vi "CRYGraph Main.vi"() -> ()   [LabVIEW 2013]
uses:
  Control/SplitterBar.ctl
  <vilib>/Utility/inputDevices.llb/closeMouse.vi
  CRYNew View Global.vi
  CRYView Global.vi
  <vilib>/Utility/inputDevices.llb/mouseAcquire.vi
  SubVI/CRYMain Sub Window Global.vi
  <vilib>/Utility/cursorutil.llb/Set Cursor (Icon Pict).vi
panel:
  in  "bWaitCommand":bool
  in  "Docking Start":bool
  in  "nIDV":i32=10
  in  "pSPRefParent":refnum<vi>
  in  "pVIRefParent":refnum<vi>
  in  "sViewName":string="DataView"
  out "Index":i32
  in  "stop":bool
  out "StateOut":bool
  out "Bar_shadow":bool
  in  "Resize FrontPanel":bool
  in  "Add Top":bool
  in  "Add Left":bool
  out "s2":T1
  out "s30":T1
  out "s29":T1
  out "s28":T1
  out "s27":T1
  out "s26":T1
  out "s25":T1
  in  "Mouse Pos":T2
  in  "ToolbarClicked":bool
  in  "Add Bottom":bool
  in  "activated_idx":i32
  in  "close_panel":bool=TRUE
  in  "Resize_Panels":bool
  in  "splitter_down_flag":bool=TRUE
  in  "spliter_index":i32
  out "s7":T1
  out "s1":T1
  out "s12":T1
  out "s5":T1
  out "s6":T1
  out "s11":T1
  out "s10":T1
  out "s19":T1
  out "s9":T1
  out "s8":T1
  out "s24":T1
  out "s23":T1
  out "s22":T1
  out "s21":T1
  out "s20":T1
  out "s18":T1
  out "s17":T1
  out "s16":T1
  out "s15":T1
  out "s14":T1
  out "s13":T1
  out "s4":T1
  out "s3":T1
  in  "Add Right":bool
types:
  T1 = typedef "SplitterBar.ctl" = bool
  T2 = cluster{"Horizontal":i32, "Vertical":i32, "Scrolling":i32}
  T3 = cluster{"Ctrl Reference":refnum<vi>, "bObjMove":bool, "Position_top":i32, "Position_objtop":i32, "isVertical":bool, "Position_left":i32, "Position_objleft":i32}
  T4 = cluster{"sAction":string, "sType":string, "sQueueName":string, "sGraphName":string, "sData":string, "nData":i32, "pVIRef":refnum<vi>, "pSPRef":refnum<vi>}
  T5 = cluster{"TitlebarActiveColor Graph":u32, "TitlebarActiveColor Graph 2":u32}[]
  T6 = typedef "Graph Main Info Cluster.ctl" = cluster{"Selected_BarIdx":i32, "Selected_PanelIdx":i32, "Graph Main VIRef":refnum<vi>, "ToolBarClick":bool, "Spliter Ref Array":refnum<vi>[], "Panel Ref Array":refnum<vi>[], "Spliter_matrix":i32[][], "Panel_matrix":i32[][], "child_spliterIdx_matrix":i32[][], "split_pos_matrix":i32[][], "Title State":bool, "sQueueName":string, "Frame nID":i32, "Graph VIRef Array":cluster{"Graph VIRef":refnum<vi>, "Panel Idx":i32, "Frame VIRef":refnum<vi>, "Icon Ring":i32, "Graph Type":string}[], "View Type":string}
  T7 = cluster{"nID":i32, "sName":string, "sType":string, "sProperty":string, "sTemplet":string, "sDocking":string, "pVIRef":refnum<vi>, "pSPRef":refnum<vi>, "pRefTemplet":refnum<vi>, "pRefSplitter":refnum<vi>[], "nPosSplitter":i32[], "pRefSP":refnum<vi>[], "nSPID":i32[], "sSPDock":string[], "nIDFrame":i32[], "nIDPanel":i32[], "nActiveFrame":i32, "nCountFrame":i32, "cFrame":cluster{"nID":i32, "sName":string, "sType":string, "sTitle":string, "sIcon":string, "pVIRef":refnum<vi>, "pSPRef":refnum<vi>, "cWin":cluster{"sName":string, "sType":string, "pVIRef":refnum<vi>, "sData":string}, "cTab":cluster{"sTitle":string, "sIcon":string, "pSpliter":refnum<vi>, "nAvtivePage":i32, "nIDPage":i32[], "nIDFrame":i32[]}, "sData":string}[], "sData":string, "sSplitterName":string[]}
  T8 = cluster{"sCmdType":string, "nIDView":i32, "sAction":string, "sData":string, "sOption":string, "nData":i32, "nOption":i32, "pVIRef":refnum<vi>, "pSPRef":refnum<vi>, "bWaitRef":refnum<vi>, "Result":variant}
  T9 = cluster{"button 1":bool, "button 2":bool, "button 3":bool, "button 4":bool}
  T10 = typedef "LVRectTypeDef.ctl" = cluster{"Left":i16, "Top":i16, "Right":i16, "Bottom":i16}
  T11 = cluster{"Left":bool, "Top":bool, "Right":bool, "Bottom":bool}
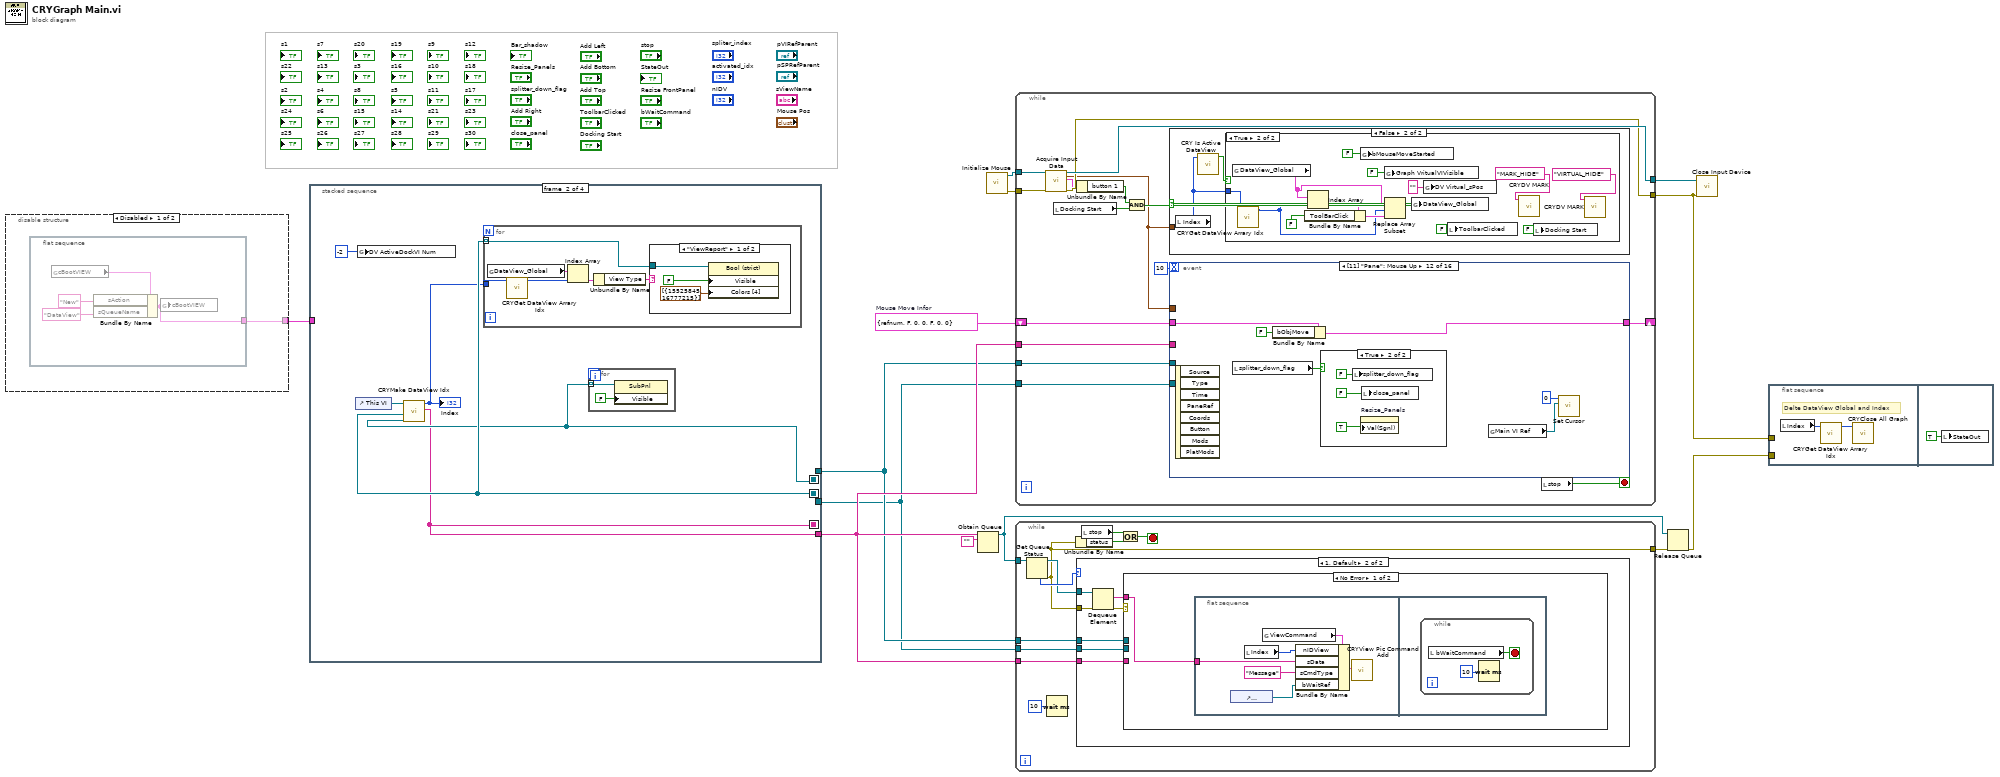
[diagram p0: block diagram]
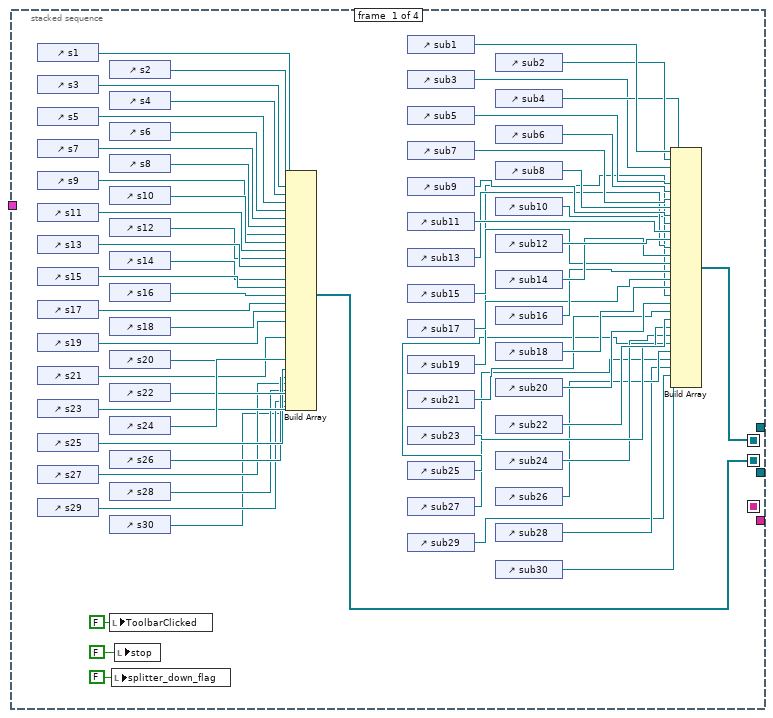
[diagram p3: hidden frame]
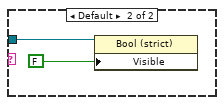
[diagram p4: hidden frame]
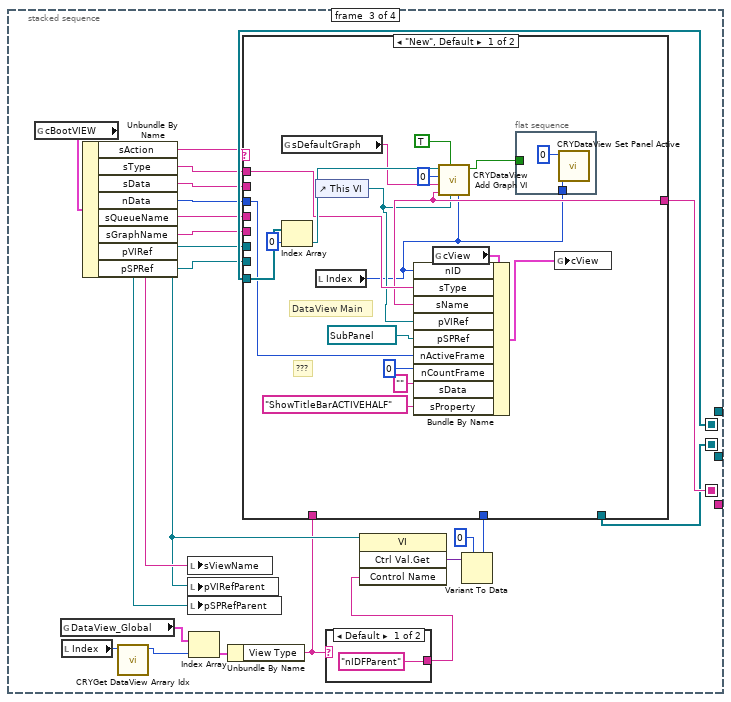
[diagram p5: hidden frame]
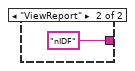
[diagram p6: hidden frame]
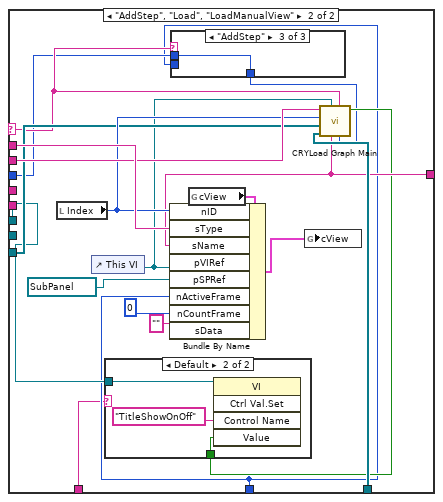
[diagram p7: hidden frame]
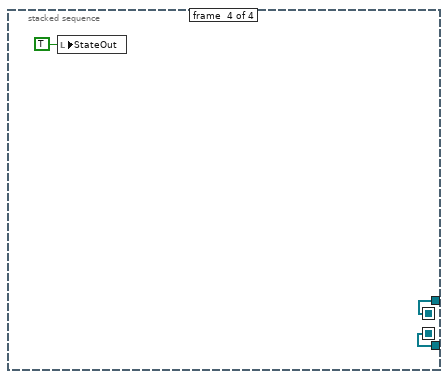
[diagram p11: hidden frame]
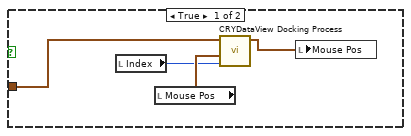
[diagram p14: hidden frame]
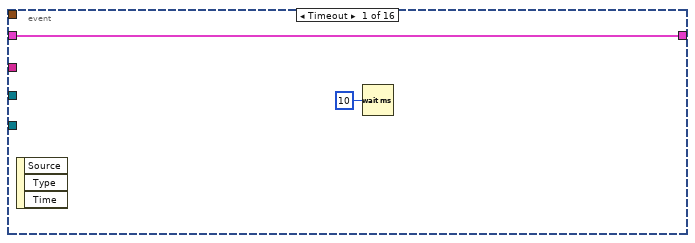
[diagram p16: hidden frame]
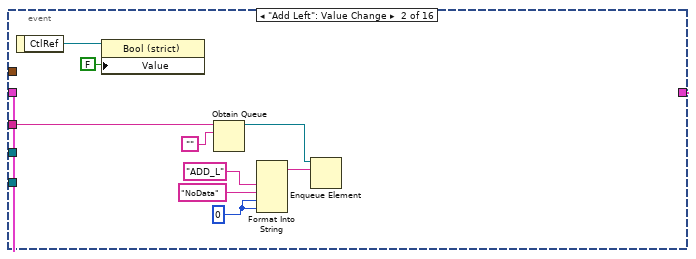
[diagram p17: hidden frame]
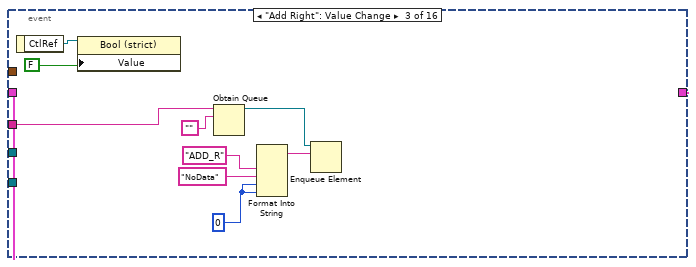
[diagram p18: hidden frame]
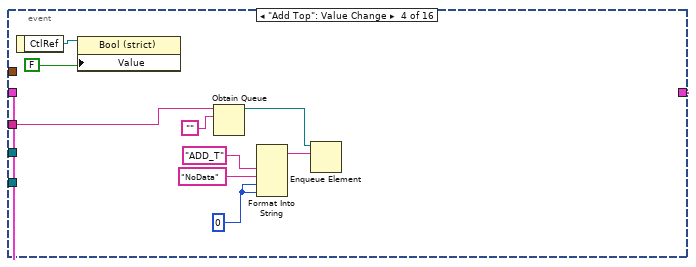
[diagram p19: hidden frame]
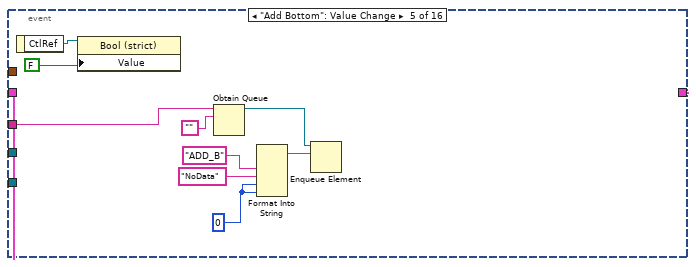
[diagram p20: hidden frame]
diagram:
  w13 = T3 {"Ctrl Reference"=refnum, "bObjMove"=FALSE, "Position_top"=0, "Position_objtop"=0, "isVertical"=FALSE, "Position_left"=0, "Position_objleft"=0}  # Mouse Move Infor
  n1 = disable-structure shown="Disabled" {
    disable-tunnel: [w14 _] -> w4
    frame Disabled {
      n2 = flat-sequence {
        tunnel: [w15] -> w14
        frame #0 {
          n3 = global read "CRYView Global.vi" "cBootVIEW"() -> (w18:T4)
          n4 = Bundle By Name(cluster=w18, "sAction"="New", "sQueueName"="DataView") -> (w15:T4)
          n5 = global write "CRYView Global.vi" "cBootVIEW"(w15) -> ()
        }
      }
    }
    frame Enabled {
    }
  }
  n6 = stacked-sequence {
    seq-local: [w22 _ _ _] -> [_ w88 w113 w171]
    seq-local: [w45 _ _ _] -> [_ w87 w122 w172]
    seq-local: [_ w86 _ _] -> [_ _ w123 _]
    tunnel: [_ w86 _ _] -> w5
    tunnel: w4 -> [_ _ _ _]
    tunnel: [_ _ _ w171] -> w1
    tunnel: [_ _ _ w172] -> w3
    frame #0 {
      n7 = control-ref of="s1"() -> (w24:refnum<vi>)
      n8 = control-ref of="s3"() -> (w46:refnum<vi>)
      n9 = control-ref of="s5"() -> (w48:refnum<vi>)
      n10 = control-ref of="s7"() -> (w50:refnum<vi>)
      n11 = control-ref of="s9"() -> (w52:refnum<vi>)
      n12 = control-ref of="s11"() -> (w54:refnum<vi>)
      n13 = control-ref of="s13"() -> (w56:refnum<vi>)
      n14 = control-ref of="s15"() -> (w58:refnum<vi>)
      n15 = control-ref of="s17"() -> (w60:refnum<vi>)
      n16 = control-ref of="s19"() -> (w62:refnum<vi>)
      n17 = control-ref of="s21"() -> (w64:refnum<vi>)
      n18 = control-ref of="s23"() -> (w66:refnum<vi>)
      n19 = control-ref of="s25"() -> (w31:refnum<vi>)
      n20 = control-ref of="s27"() -> (w29:refnum<vi>)
      n21 = control-ref of="s29"() -> (w27:refnum<vi>)
      n22 = control-ref of="s2"() -> (w23:refnum<vi>)
      n23 = control-ref of="s4"() -> (w47:refnum<vi>)
      n24 = control-ref of="s6"() -> (w49:refnum<vi>)
      n25 = control-ref of="s8"() -> (w51:refnum<vi>)
      n26 = control-ref of="s10"() -> (w53:refnum<vi>)
      n27 = control-ref of="s12"() -> (w55:refnum<vi>)
      n28 = control-ref of="s14"() -> (w57:refnum<vi>)
      n29 = control-ref of="s16"() -> (w59:refnum<vi>)
      n30 = control-ref of="s18"() -> (w61:refnum<vi>)
      n31 = control-ref of="s20"() -> (w63:refnum<vi>)
      n32 = control-ref of="s22"() -> (w65:refnum<vi>)
      n33 = control-ref of="s24"() -> (w67:refnum<vi>)
      n34 = control-ref of="s26"() -> (w30:refnum<vi>)
      n35 = control-ref of="s28"() -> (w28:refnum<vi>)
      n36 = control-ref of="s30"() -> (w26:refnum<vi>)
      n37 = local write "ToolbarClicked"(FALSE ("ToolbarClicked")) -> ()
      n38 = local write "splitter_down_flag"(FALSE ("m_down_flag")) -> ()
      n39 = local write "stop"(FALSE ("stop")) -> ()
      n40 = Build Array(w24, w23, w46, w47, w48, w49, w50, w51, w52, w53, w54, w55, w56, w57, w58, w59, w60, w61, w62, w63, w64, w65, w66, w67, w31, w30, w29, w28, w27, w26) -> (w22:refnum<vi>[])
      n41 = control-ref of="sub1"() -> (w83:refnum<vi>)
      n42 = control-ref of="sub3"() -> (w25:refnum<vi>)
      n43 = control-ref of="sub5"() -> (w80:refnum<vi>)
      n44 = control-ref of="sub7"() -> (w78:refnum<vi>)
      n45 = control-ref of="sub9"() -> (w76:refnum<vi>)
      n46 = control-ref of="sub11"() -> (w75:refnum<vi>)
      n47 = control-ref of="sub13"() -> (w73:refnum<vi>)
      n48 = control-ref of="sub15"() -> (w71:refnum<vi>)
      n49 = control-ref of="sub17"() -> (w69:refnum<vi>)
      n50 = control-ref of="sub19"() -> (w43:refnum<vi>)
      n51 = control-ref of="sub21"() -> (w41:refnum<vi>)
      n52 = control-ref of="sub23"() -> (w39:refnum<vi>)
      n53 = control-ref of="sub25"() -> (w37:refnum<vi>)
      n54 = control-ref of="sub27"() -> (w35:refnum<vi>)
      n55 = control-ref of="sub29"() -> (w33:refnum<vi>)
      n56 = control-ref of="sub2"() -> (w82:refnum<vi>)
      n57 = control-ref of="sub4"() -> (w81:refnum<vi>)
      n58 = control-ref of="sub6"() -> (w79:refnum<vi>)
      n59 = control-ref of="sub8"() -> (w77:refnum<vi>)
      n60 = control-ref of="sub10"() -> (w68:refnum<vi>)
      n61 = control-ref of="sub12"() -> (w74:refnum<vi>)
      n62 = control-ref of="sub14"() -> (w72:refnum<vi>)
      n63 = control-ref of="sub16"() -> (w70:refnum<vi>)
      n64 = control-ref of="sub18"() -> (w44:refnum<vi>)
      n65 = control-ref of="sub20"() -> (w42:refnum<vi>)
      n66 = control-ref of="sub22"() -> (w40:refnum<vi>)
      n67 = control-ref of="sub24"() -> (w38:refnum<vi>)
      n68 = control-ref of="sub26"() -> (w36:refnum<vi>)
      n69 = control-ref of="sub28"() -> (w34:refnum<vi>)
      n70 = control-ref of="sub30"() -> (w32:refnum<vi>)
      n71 = Build Array(w83, w82, w25, w81, w80, w79, w78, w77, w76, w68, w75, w74, w73, w72, w71, w70, w69, w44, w43, w42, w41, w40, w39, w38, w37, w36, w35, w34, w33, w32) -> (w45:refnum<vi>[])
    }
    frame #1 {
      n72 = control-ref of="This VI"() -> (w89:refnum<vi>)
      n73 = global write "CRYNew View Global.vi" "DV ActiveDockVI Num"(-2 ("DV ActiveDockVI Num")) -> ()
      n74 = call "CRYMake DataView Idx.vi"("Panel Ref Array"=w87, "Spliter Ref Array"=w88, "VI Ref"=w89) -> ("sQueueName Out"=w86:string, "New DataView Idx"=w85:i32)  [unwired: 7 in]
      "Index" <- w85
      n75 = for {
        tunnel: w88 -> [w97] mode=indexing
        tunnel: w85 -> [w93]
        n76 = global read "CRYNew View Global.vi" "DataView_Global"() -> (w96:T6[])
        n77 = call "CRYGet DataView Arrary Idx.vi"("DataView Idx In"=w93) -> ("DataView Arrary Idx out"=w94:i32)  [unwired: 10 in]
        n78 = Index Array(array=w96, index=w94) -> (element=w95:T6)
        n79 = Unbundle By Name(w95) -> ("View Type"=w92:string)
        n80 = case shown="\"ViewReport\"" w92 {
          tunnel: w97 -> [w99 w101]
          frame "ViewReport" {
            n81 = property class="Bool (strict)"(reference=w99, "Visible"=FALSE, "Colors [4]"=T5 [{"TitlebarActiveColor Graph"=15525845, "TitlebarActiveColor Graph 2"=16777215}]) -> ()  [unwired: 1 in, 2 out]
          }
          frame Default {
            n82 = property class="Bool (strict)"(reference=w101, "Visible"=FALSE) -> ()  [unwired: 1 in, 2 out]
          }
        }
      }
      n83 = for {
        tunnel: w87 -> [w90] mode=indexing
        n84 = property class="SubPnl"(reference=w90, "Visible"=FALSE) -> ()  [unwired: 1 in, 2 out]
      }
    }
    frame #2 {
      n85 = global read "CRYView Global.vi" "cBootVIEW"() -> (w121:T4)
      n86 = global read "CRYNew View Global.vi" "DataView_Global"() -> (w108:T6[])
      n87 = local read "Index"() -> (w107:i32)
      n88 = Unbundle By Name(w121) -> ("sAction"=w117:string, "sType"=w116:string, "sData"=w119:string, "nData"=w118:i32, "sQueueName"=w115:string, "sGraphName"=w120:string, "pVIRef"=w109:refnum<vi>, "pSPRef"=w114:refnum<vi>)
      n89 = call "CRYGet DataView Arrary Idx.vi"("DataView Idx In"=w107) -> ("DataView Arrary Idx out"=w103:i32)  [unwired: 10 in]
      n90 = local write "sViewName"(w115) -> ()
      n91 = local write "pVIRefParent"(w109) -> ()
      n92 = local write "pSPRefParent"(w114) -> ()
      n93 = Index Array(array=w108, index=w103) -> (element=w106:T6)
      n94 = Unbundle By Name(w106) -> ("View Type"=w104:string)
      n95 = case shown="Default" w104 {
        tunnel: ["nIDFParent" ("Control Name") "nIDF" ("Control Name")] -> w105
        frame Default {
        }
        frame "ViewReport" {
        }
      }
      n96 = invoke class="VI" method="Ctrl Val.Get"(reference=w109, "Control Name"=w105) -> ("Get Control Value Variant"=w112:variant)  [unwired: 2 in, 3 out]
      n97 = Variant To Data(type=0 ("nIDFParent"), Variant=w112) -> (data=w110:i32)  [unwired: 1 in, 1 out]
      n98 = case shown="\"New\", Default" w117 {
        selector: w117 -> [_ w151]
        tunnel: w115 -> [_ _]
        tunnel: w120 -> [_ _]
        tunnel: w119 -> [_ w158]
        tunnel: w118 -> [w127 w150]
        tunnel: w109 -> [_ w148]
        tunnel: w114 -> [_ _]
        tunnel: w116 -> [w133 w164]
        tunnel: w123 -> [w132 w153]
        tunnel: w122 -> [w143 w156]
        tunnel: w113 -> [_ w155]
        tunnel: w110 -> [_ w147]
        tunnel: w104 -> [_ w146]
        frame "New", Default {
          # "DataView Main"
          # "???"
          n99 = global read "CRYView Global.vi" "sDefaultGraph"() -> (w134:string)
          n100 = Index Array(array=w143, index=0) -> (element=w141:refnum<vi>)
          n101 = control-ref of="This VI"() -> (w129:refnum<vi>)
          n102 = local read "Index"() -> (w126:i32)
          n103 = global read "CRYView Global.vi" "cView"() -> (w135:T7)
          n104 = Bundle By Name(cluster=w135, "nID"=w126, "sType"=w133, "sName"=w132, "pVIRef"=w129, "pSPRef"=refnum<vi> refnum, "nActiveFrame"=w127, "nCountFrame"=0 ("nActiveFrame"), "sData"="", "sProperty"="ShowTitleBarACTIVEHALF") -> (w130:T7)
          n105 = call "CRYDataView Add Graph VI.vi"("DataView Idx"=w126, "Graph Main VIRef In"=w129, "isFirstPanel"=TRUE, "Queue Name"=w132, "GraphType"=w134, "panel_index"=0, "Panel Ref In"=w141) -> ("bResult"=w128:bool)  [unwired: 4 in]
          n106 = flat-sequence {
            tunnel: w126 -> [w145]
            tunnel: w128 -> [_]
            frame #0 {
              n107 = call "CRYDataView Set Panel Active.vi"("DataView Index"=w145, "Selected Panel Idx In"=0) -> ()  [unwired: 10 in]
            }
          }
          n108 = global write "CRYView Global.vi" "cView"(w130) -> ()
        }
        frame "AddStep", "Load", "LoadManualView" {
          n109 = local read "Index"() -> (w157:i32)
          n110 = control-ref of="This VI"() -> (w154:refnum<vi>)
          n111 = case shown="\"AddStep\"" w151 {
            tunnel: w147 -> [_ w169 _]
            tunnel: [w168 w169 w170] -> w149
            tunnel: w150 -> [w168 _ w170]
            frame "LoadManualView", Default {
            }
            frame "Load" {
            }
            frame "AddStep" {
            }
          }
          n112 = global read "CRYView Global.vi" "cView"() -> (w163:T7)
          n113 = Bundle By Name(cluster=w163, "nID"=w157, "sType"=w164, "sName"=w153, "pVIRef"=w154, "pSPRef"=refnum<vi> refnum, "nActiveFrame"=w147, "nCountFrame"=0 ("nActiveFrame"), "sData"="") -> (w159:T7)
          n114 = global write "CRYView Global.vi" "cView"(w159) -> ()
          n115 = call "CRYLoad Graph Main.vi"("nData"=w149, "sAction"=w151, "sQueue Name"=w153, "Graph Main Ref"=w154, "Spliter Ref Array"=w155, "Panel Ref Array"=w156, "DataView Index"=w157, "Flattend Data"=w158) -> ("Title State"=w152:bool)  [unwired: 3 in]
          n116 = case shown="Default" w146 {
            tunnel: w152 -> [_ w166]
            tunnel: w148 -> [_ w165]
            frame "ViewReport" {
            }
            frame Default {
              n117 = invoke class="VI" method="Ctrl Val.Set"(reference=w165, "Control Name"="TitleShowOnOff" ("Resize Panel Str"), "Value"=w166) -> ()  [unwired: 2 in, 5 out]
            }
          }
        }
      }
    }
    frame #3 {
      n118 = local write "StateOut"(TRUE ("StateOut")) -> ()
    }
  }
  n119 = Obtain Queue(name (unnamed)=w5, element data type="") -> (queue out=w11:refnum<queue>)  [unwired: 3 in, 2 out]
  n120 = call <vilib>:"Initialize Mouse.vi"() -> ("error out"=w9:errorcluster, "device ID"=w10:refnum<k1>)  [unwired: 10 in]
  n121 = while {
    tunnel: w11 -> [w183]
    tunnel: w1 -> [w180]
    tunnel: w3 -> [w179]
    tunnel: [w178] -> w7
    tunnel: w5 -> [w174]
    stop <- w175 stop-if-true
    n122 = Get Queue Status(queue=w183) -> (queue out=w181:refnum<queue>, error out=w178:errorcluster, # elements in queue=w182:i32)  [unwired: 2 in, 5 out]
    n123 = Wait (ms)(milliseconds to wait=u32 10) -> ()  [unwired: 1 out]
    n124 = Unbundle By Name(w178) -> ("status"=w177:bool)
    n125 = case shown="1, Default" w182 {
      tunnel: w178 -> [_ w187]
      tunnel: w181 -> [_ w191]
      tunnel: w180 -> [_ w189]
      tunnel: w179 -> [_ w188]
      tunnel: w174 -> [_ w185]
      frame 0 {
      }
      frame 1, Default {
        n126 = Dequeue Element(queue=w191, error in (no error)=w187) -> (element=w190:string, error out=w186:errorcluster)  [unwired: 1 in, 2 out]
        n127 = case shown="No Error" w186 {
          tunnel: w190 -> [w192 _]
          tunnel: w189 -> [_ _]
          tunnel: w188 -> [_ _]
          tunnel: w185 -> [_ _]
          frame No Error {
            n128 = flat-sequence {
              tunnel: w192 -> [w196]
              frame #0 {
                n129 = control-ref of="bWaitCommand"() -> (w195:refnum<vi>)
                n130 = local read "Index"() -> (w193:i32)
                n131 = global read "CRYView Global.vi" "ViewCommand"() -> (w194:T8)
                n132 = Bundle By Name(cluster=w194, "nIDView"=w193, "sData"=w196, "sCmdType"="Message" ("sAction"), "bWaitRef"=w195) -> (w197:T8)
                n133 = call "CRYView Pic Command Add.vi"("cCommand"=w197) -> ()  [unwired: 11 in]
              }
              frame #1 {
                n134 = while {
                  stop <- w200 stop-if-true
                  n135 = local read "bWaitCommand"() -> (w200:bool)
                  n136 = Wait (ms)(milliseconds to wait=u32 10) -> ()  [unwired: 1 out]
                }
              }
            }
          }
          frame Error {
          }
        }
      }
    }
    n137 = local read "stop"() -> (w176:bool)
    n138 = Or(x=w176, y=w177) -> (x .or. y?=w175:bool)
  }
  n139 = while {
    tunnel: w3 -> [w202]
    shift-right: [w214] -> _
    shift-left: w13 -> [w216]
    tunnel: w1 -> [w215]
    tunnel: w5 -> [w213]
    tunnel: w10 -> [w212]
    tunnel: w9 -> [w211]
    tunnel: [w210] -> w8
    tunnel: [w209] -> w2
    stop <- w201 stop-if-true
    n140 = call-poly <vilib>:"Acquire Input Data.vi"("device ID"=w212, "error in (no error)"=w211) -> ("device ID"=w210:refnum<k1>, "axis info"=w203:T2, "button info"=w208:T9, "error out"=w209:errorcluster)  [unwired: 14 in]
    n141 = local read "Docking Start"() -> (w206:bool)
    n142 = Unbundle By Name(w208) -> ("button 1"=w205:bool)
    n143 = And(x=w205, y=w206) -> (x .and. y?=w204:bool)
    n144 = case shown="False" w204 {
      tunnel: w203 -> [w220 _]
      frame True {
        n145 = local read "Index"() -> (w217:i32)
        n146 = local read "Mouse Pos"() -> (w219:T2)
        n147 = call "CRYDataView Docking Process.vi"("DataView Index"=w217, "Start Pos"=w219, "Mouse Pos"=w220) -> ("StartPositin Out"=w218:T2)  [unwired: 8 in]
        n148 = local write "Mouse Pos"(w218) -> ()
      }
      frame False {
        n149 = local read "Index"() -> (w222:i32)
        n150 = call "CRY Is Active DataView.vi"("DataView Index"=w222) -> ("bResult"=w221:bool)  [unwired: 10 in]
        n151 = case shown="True" w221 {
          tunnel: w222 -> [_ w227]
          frame False {
          }
          frame True {
            n152 = global read "CRYNew View Global.vi" "DataView_Global"() -> (w232:T6[])
            n153 = call "CRYGet DataView Arrary Idx.vi"("DataView Idx In"=w227) -> ("DataView Arrary Idx out"=w226:i32)  [unwired: 10 in]
            n154 = Index Array(array=w232, index=w226) -> (element=w235:T6)
            n155 = Bundle By Name(cluster=w235, "ToolBarClick"=FALSE) -> (w234:T6)
            n156 = global write "CRYNew View Global.vi" "bMouseMoveStarted"(FALSE ("VritualVIVisible")) -> ()
            n157 = global write "CRYNew View Global.vi" "Graph VritualVIVisible"(FALSE ("VritualVIVisible")) -> ()
            n158 = Replace Array Subset(array=w232, new element=w234, index=w226) -> (w236:T6[])
            n159 = global write "CRYNew View Global.vi" "DataView_Global"(w236) -> ()
            n160 = global write "CRYNew View Global.vi" "DV Virtual_sPos"("" ("DV Virtual_sPos")) -> ()
            n161 = local write "ToolbarClicked"(FALSE ("ToolbarClicked")) -> ()
            n162 = call "CRYDV MARK.vi"("sAction"="MARK_HIDE") -> ()  [unwired: 9 in, 1 out]
            n163 = local write "Docking Start"(FALSE ("Docking Start")) -> ()
            n164 = call "CRYDV MARK.vi"("sAction"="VIRTUAL_HIDE") -> ()  [unwired: 9 in, 1 out]
          }
        }
      }
    }
    n165 = event shown="[11] \"Pane\": Mouse Up" {
      selector: _ -> [_ _ _ _ _ _ _ _ _ _ _ _ _ _ _ _]
      dyn-events: _ -> [_ _ _ _ _ _ _ _ _ _ _ _ _ _ _ _]
      timeout: 10 -> [_ _ _ _ _ _ _ _ _ _ _ _ _ _ _ _]
      tunnel: w202 -> [_ _ _ _ _ _ _ _ _ w291 _ _ _ _ _ _]
      tunnel: w216 -> [w237 w246 w256 w266 w276 w281 w284 w288 _ _ w306 w313 w322 w338 _ _]
      tunnel: [w237 w246 w256 w266 w276 w281 w284 w288 _ _ w305 w315 w324 w339 _ _] -> w214
      tunnel: w215 -> [_ _ _ _ _ _ _ _ _ _ _ _ _ _ _ _]
      tunnel: w213 -> [_ w239 w249 w259 w269 _ _ _ _ _ _ _ _ w331 _ _]
      tunnel: w203 -> [_ _ _ _ _ _ _ w287 w289 w292 w307 _ _ _ _ _]
      event Timeout {
        n166 = event-data() -> ()  [unwired: 1 in, 3 out]
        n167 = Wait (ms)(milliseconds to wait=u32 10) -> ()  [unwired: 1 out]
      }
      event "Add Left": Value Change {
        w240 = 0 ("input 3")
        n168 = event-data() -> ("CtlRef"=w248:refnum<vi>)  [unwired: 1 in]
        n169 = property class="Bool (strict)"(reference=w248, "Value"=FALSE) -> ()  [unwired: 1 in, 2 out]
        n170 = Obtain Queue(name (unnamed)=w239, element data type="") -> (queue out=w242:refnum<queue>)  [unwired: 3 in, 2 out]
        n171 = Format Into String("ADD_L" ("input 1"), "NoData" ("input 2"), w240, w240) -> (resulting string=w241:string)  [unwired: 3 in, 1 out]
        n172 = Enqueue Element(queue=w242, element=w241) -> ()  [unwired: 1 in, 4 out]
      }
      event "Add Right": Value Change {
        w250 = 0 ("input 3")
        n173 = event-data() -> ("CtlRef"=w258:refnum<vi>)  [unwired: 1 in]
        n174 = property class="Bool (strict)"(reference=w258, "Value"=FALSE) -> ()  [unwired: 1 in, 2 out]
        n175 = Obtain Queue(name (unnamed)=w249, element data type="") -> (queue out=w252:refnum<queue>)  [unwired: 3 in, 2 out]
        n176 = Format Into String("ADD_R" ("input 1"), "NoData" ("input 2"), w250, w250) -> (resulting string=w251:string)  [unwired: 3 in, 1 out]
        n177 = Enqueue Element(queue=w252, element=w251) -> ()  [unwired: 1 in, 4 out]
      }
      event "Add Top": Value Change {
        w260 = 0 ("input 3")
        n178 = event-data() -> ("CtlRef"=w268:refnum<vi>)  [unwired: 1 in]
        n179 = property class="Bool (strict)"(reference=w268, "Value"=FALSE) -> ()  [unwired: 1 in, 2 out]
        n180 = Obtain Queue(name (unnamed)=w259, element data type="") -> (queue out=w262:refnum<queue>)  [unwired: 3 in, 2 out]
        n181 = Format Into String("ADD_T" ("input 1"), "NoData" ("input 2"), w260, w260) -> (resulting string=w261:string)  [unwired: 3 in, 1 out]
        n182 = Enqueue Element(queue=w262, element=w261) -> ()  [unwired: 1 in, 4 out]
      }
      event "Add Bottom": Value Change {
        w270 = 0 ("input 3")
        n183 = event-data() -> ("CtlRef"=w278:refnum<vi>)  [unwired: 1 in]
        n184 = property class="Bool (strict)"(reference=w278, "Value"=FALSE) -> ()  [unwired: 1 in, 2 out]
        n185 = Obtain Queue(name (unnamed)=w269, element data type="") -> (queue out=w272:refnum<queue>)  [unwired: 3 in, 2 out]
        n186 = Format Into String("ADD_B" ("input 1"), "NoData" ("input 2"), w270, w270) -> (resulting string=w271:string)  [unwired: 3 in, 1 out]
        n187 = Enqueue Element(queue=w272, element=w271) -> ()  [unwired: 1 in, 4 out]
      }
      event Mouse Enter {
        # "Splitter Mouse Enter"
        n188 = event-data() -> ()  [unwired: 1 in, 4 out]
        n189 = global read "CRYMain Sub Window Global.vi" "Main VI Ref"() -> (w279:refnum<vi>)
        n190 = call-poly <vilib>:"Set Cursor.vi"("VI reference (current VI)"=w279, "icon"=u16 6) -> ()  [unwired: 1 in, 9 out]
      }
      event Mouse Leave {
        # "Splitter Mouse Leave"
        n191 = event-data() -> ()  [unwired: 1 in, 4 out]
        n192 = global read "CRYMain Sub Window Global.vi" "Main VI Ref"() -> (w282:refnum<vi>)
        n193 = call-poly <vilib>:"Set Cursor.vi"("VI reference (current VI)"=w282, "icon"=u16 0) -> ()  [unwired: 1 in, 9 out]
      }
      event Mouse Move {
        n194 = event-data() -> ()  [unwired: 1 in, 5 out]
        n195 = control-ref of="Bar_shadow"() -> (w286:refnum<vi>)
        n196 = local read "Index"() -> (w285:i32)
        n197 = call "CRYDataView SplitterShadow Moving Process.vi"("DataView Index"=w285, "Bar_shadow ref"=w286, "Mouse Pos"=w287, "SpliterMoveInfo"=w288) -> ()  [unwired: 8 in]
      }
      event Mouse Down {
        n198 = event-data() -> ()  [unwired: 1 in, 6 out]
        n199 = local write "Mouse Pos"(w289) -> ()
      }
      event "ToolbarClicked": Value Change {
        n200 = event-data() -> ("NewVal"=w290:bool)  [unwired: 1 in, 5 out]
        n201 = case shown="True" w290 {
          tunnel: w292 -> [_ _]
          tunnel: w291 -> [_ w293]
          frame False {
          }
          frame True {
            n202 = stacked-sequence {
              tunnel: w293 -> [w300 _]
              frame #0 {
                n203 = global read "CRYNew View Global.vi" "DataView_Global"() -> (w302:T6[])
                n204 = local read "Index"() -> (w295:i32)
                n205 = call "CRYGet DataView Arrary Idx.vi"("DataView Idx In"=w295) -> ("DataView Arrary Idx out"=w294:i32)  [unwired: 10 in]
                n206 = Index Array(array=w302, index=w294) -> (element=w301:T6)
                n207 = Unbundle By Name(w301) -> ("Selected_PanelIdx"=w299:i32)
                n208 = Index Array(array=w300, index=w299) -> (element=w298:refnum<vi>)
                n209 = property class="SubPnl"(reference=w298) -> ("InsertedVI"=w297:refnum<vi>)  [unwired: 1 in, 2 out]
                n210 = property class="VI"(reference=w297) -> ("Front Panel.PanelBounds"=w296:T10)  [unwired: 1 in, 2 out]
                n211 = global write "CRYNew View Global.vi" "Graph VritualBounds"(w296) -> ()
              }
              frame #1 {
                n212 = local write "Docking Start"(TRUE ("Docking Start")) -> ()
              }
            }
          }
        }
      }
      event Mouse Down {
        # "Splitter Mouse down"
        n213 = event-data() -> ("CtlRef"=w304:refnum<vi>)  [unwired: 1 in, 5 out]
        n214 = control-ref of="Bar_shadow"() -> (w310:refnum<vi>)
        n215 = local read "Index"() -> (w308:i32)
        n216 = call "CRYDataView Splitter MDown Process.vi"("DataView Index"=w308, "Selected Spliter Ref"=w304, "Bar_shadow ref"=w310, "Mouse Pos"=w307, "SpliterMove Info"=w306) -> ("SpliterMove Out"=w305:T3)  [unwired: 6 in]
        n217 = local write "splitter_down_flag"(TRUE ("m_down_flag")) -> ()
      }
      event Mouse Up {
        n218 = event-data() -> ()  [unwired: 1 in, 8 out]
        n219 = local read "splitter_down_flag"() -> (w314:bool)
        n220 = Bundle By Name(cluster=w313, "bObjMove"=FALSE ("객체이동")) -> (w315:T3)
        n221 = case shown="True" w314 {
          frame False {
          }
          frame True {
            n222 = local write "splitter_down_flag"(FALSE ("m_down_flag")) -> ()
            n223 = property on="Resize_Panels" class="Bool (strict)"("Val(Sgnl)"=TRUE ("Value (Signaling)")) -> ()  [unwired: 2 in, 2 out]
            n224 = local write "close_panel"(FALSE ("close_panel")) -> ()
          }
        }
        n225 = global read "CRYMain Sub Window Global.vi" "Main VI Ref"() -> (w311:refnum<vi>)
        n226 = call-poly <vilib>:"Set Cursor.vi"("VI reference (current VI)"=w311, "icon"=u16 0) -> ()  [unwired: 1 in, 9 out]
      }
      event Mouse Leave {
        n227 = event-data() -> ()  [unwired: 1 in, 4 out]
        n228 = local read "splitter_down_flag"() -> (w323:bool)
        n229 = Bundle By Name(cluster=w322, "bObjMove"=FALSE ("객체이동")) -> (w324:T3)
        n230 = case shown="True" w323 {
          frame False {
          }
          frame True {
            n231 = local write "splitter_down_flag"(FALSE ("m_down_flag")) -> ()
            n232 = local write "close_panel"(FALSE ("close_panel")) -> ()
            n233 = property on="Resize_Panels" class="Bool (strict)"("Val(Sgnl)"=TRUE ("Value (Signaling)")) -> ()  [unwired: 2 in, 2 out]
          }
        }
        n234 = global read "CRYMain Sub Window Global.vi" "Main VI Ref"() -> (w320:refnum<vi>)
        n235 = call-poly <vilib>:"Set Cursor.vi"("VI reference (current VI)"=w320, "icon"=u16 0) -> ()  [unwired: 1 in, 9 out]
      }
      event "Resize_Panels": Value Change {
        n236 = event-data() -> ()  [unwired: 1 in, 6 out]
        n237 = Bundle By Name(cluster=w338, "bObjMove"=FALSE ("객체이동")) -> (w339:T3)
        n238 = local read "Index"() -> (w330:i32)
        n239 = Obtain Queue(name (unnamed)=w331, element data type="") -> (queue out=w335:refnum<queue>)  [unwired: 3 in, 2 out]
        n240 = Format Into String("GRAPH_MAIN_SUBPANEL_RESIZE" ("input 1"), "NoData" ("input 2"), 0 ("input 3"), w330) -> (resulting string=w336:string)  [unwired: 3 in, 1 out]
        n241 = local write "Resize_Panels"(FALSE ("Resize_Panels")) -> ()
        n242 = Enqueue Element(queue=w335, element=w336) -> ()  [unwired: 1 in, 4 out]
        n243 = disable-structure shown="Disabled" {
          frame Disabled {
            n244 = call-poly <vilib>:"Set Cursor.vi"("icon"=u16 1) -> ()  [unwired: 2 in, 9 out]
          }
          frame Enabled {
          }
        }
      }
      event Pane Size {
        # "???????????????"
        n245 = event-data() -> ("OldBnds"=w349:T10, "NewBnds"=w348:T10)  [unwired: 1 in, 4 out]
        n246 = Equal?(x=w349, y=w348) -> (x = y?=w347:T11)
        n247 = Unbundle By Name(w347) -> ("Left"=w346:bool, "Top"=w345:bool, "Right"=w344:bool, "Bottom"=w343:bool)
        n248 = property on="Resize FrontPanel" class="Bool (strict)"("Val(Sgnl)"=TRUE ("Value (Signaling)")) -> ()  [unwired: 2 in, 2 out]
        n249 = Compound Arithmetic op=AND(w346, w345, w344, w343) -> ()  [unwired: 1 out]
      }
      event "Resize FrontPanel": Value Change {
        n250 = event-data() -> ()  [unwired: 1 in, 6 out]
        n251 = local read "Index"() -> (w350:i32)
        n252 = control-ref of="This VI"() -> (w351:refnum<vi>)
        n253 = local write "Resize FrontPanel"(FALSE ("Resize FrontPanel")) -> ()
        n254 = call "CRYDataView Pane Resize Proc.vi"("DataView Index"=w350, "VI Ref"=w351) -> ()  [unwired: 10 in]
      }
    }
    n255 = local read "stop"() -> (w201:bool)
  }
  n256 = Release Queue(queue=w11, error in (no error)=w7) -> (error out=w6:errorcluster)  [unwired: 1 in, 2 out]
  n257 = call-poly <vilib>:"Close Input Device.vi"("error in (no error)"=w2, "device ID"=w8) -> ()  [unwired: 8 in, 1 out]
  n258 = flat-sequence {
    tunnel: w6 -> [_]
    tunnel: w2 -> [_]
    frame #0 {
      # "Delte DataView Global and Index"
      n259 = local read "Index"() -> (w353:i32)
      n260 = call "CRYGet DataView Arrary Idx.vi"("DataView Idx In"=w353) -> ("DataView Arrary Idx out"=w354:i32)  [unwired: 10 in]
      n261 = call "CRYClose All Graph.vi"("DataView Array Idx In"=w354) -> ()  [unwired: 11 in]
    }
    frame #1 {
      n262 = local write "StateOut"(TRUE ("StateOut")) -> ()
    }
  }
